vi "NI VeriStand - Pointer to Item Reference.vi"(8 "error in (no error)":errorcluster, 10 "Node Pointer":T1) -> (0 "error out":errorcluster, 3 "Item Ref out":T2 format="%.0x")   [LabVIEW 2020, in "Custom Device API.lvlib"]
doc: "Converts a pointer to a node in the system definition file into an item reference for the same node. You can use this VI to switch from the System Explorer .NET API to the Custom Device API VIs available in LabVIEW. The .NET API uses pointers to nodes. The LabVIEW VIs use references to items."
uses:
  <vilib>/NI VeriStand/Custom Device API/Custom Device API.lvlib
  <vilib>/NI VeriStand/Custom Device API/Custom Device Item Ref.ctl
  <vilib>/NI VeriStand/Custom Device API/Custom Device Pointer.ctl
  NationalInstruments.VeriStand.SystemStorage
  85a83d37-17bc-4dd9-8f32-bd30eae3b6af.vi
  <vilib>/NI VeriStand/Custom Device API/Custom Device Offline Path.vi
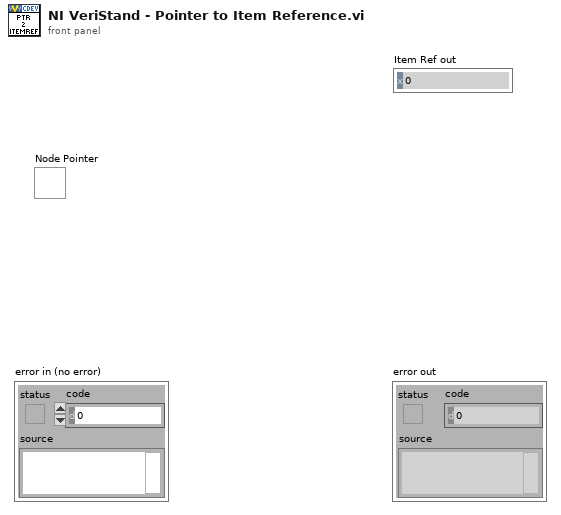
[diagram p1: front panel]
types:
  T1 = typedef "Custom Device API.lvlib/Custom Device Pointer.ctl" = refnum<k24>
  T2 = typedef "Custom Device API.lvlib/Custom Device Item Ref.ctl" = u64
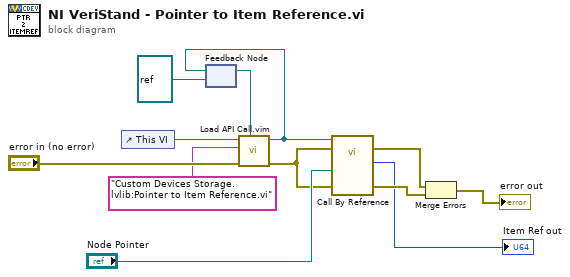
[diagram p0: block diagram]
diagram:
  n1 = control-ref of="This VI"() -> (w7:refnum<vi>)
  n2 = feedback #1(refnum<vi> refnum ("type specifier VI Refnum (for type only)")) -> (w8:refnum<vi>)
  n3 = call "Load API Call.vim"("VI reference in"=w8, "error in (no error)"="error in (no error)", "VI qualified name"="Custom Devices Storage.lvlib:Pointer to Item Reference.vi", "Caller VI ref"=w7) -> ("error out"=w5:errorcluster, "VI reference"=w4:refnum<vi>)  [unwired: 6 in]
  n4 = feedback-in #1(w4) -> ()
  n5 = call-by-ref "?"(reference=w4, error in=w5, 8:"error in (no error)"=w5, "Node"="Node Pointer") -> (error out=w1:errorcluster, 0:"error out"=w12:errorcluster, "Item Reference"=→"Item Ref out":u64)  [unwired: 8 in, 1 out]
  n6 = Merge Errors(w1, w12) -> (→"error out":errorcluster)
